vi "Tester.vi"() -> ()   [LabVIEW 2018, in "AE75TX Actor.lvlib" / "AE75TX.lvclass"]
uses:
  AE75TX.lvclass
  <vilib>/ORNL/CSEISMIC DDS/CSEISMIC DDS Base/Data Types/IED_Status.ctl
  <vilib>/ORNL/CSEISMIC DDS/CSEISMIC DDS Base/Data Types/Controls/DeviceID.ctl
  <vilib>/ORNL/CSEISMIC DDS/CSEISMIC DDS Base/Data Types/Controls/Timestamp.ctl
  <vilib>/ORNL/CSEISMIC DDS/CSEISMIC DDS Base/Data Types/DER_Measurement.ctl
  <vilib>/ORNL/CSEISMIC DDS/CSEISMIC DDS Base/Data Types/DER_Status.ctl
  <vilib>/ORNL/CSEISMIC DDS/CSEISMIC DDS Base/Data Types/Controls/DroopCurve.ctl
  Controls/PV State Selector.ctl
  Controls/Modbus Configuration Cluster.ctl
  Controls/Scaling Coefficients Measurements.ctl
  <vilib>/Modbus/master/Create Master Instance (TCP).vi
  <vilib>/Modbus/master/Modbus Master.lvclass
  <vilib>/ORNL/CSEISMIC DDS/CSEISMIC DDS Base/CSEISMIC DDS.lvclass
panel:
  in  "Ramp Rate (kVA/s)":u16
  in  "Curtailment (%)":u16
  in  "Write Curtailment":bool
  out "DER_Status":T1
  out "DER_Measurement":T4
  out "IED_Status":T5
  in  "stop":bool
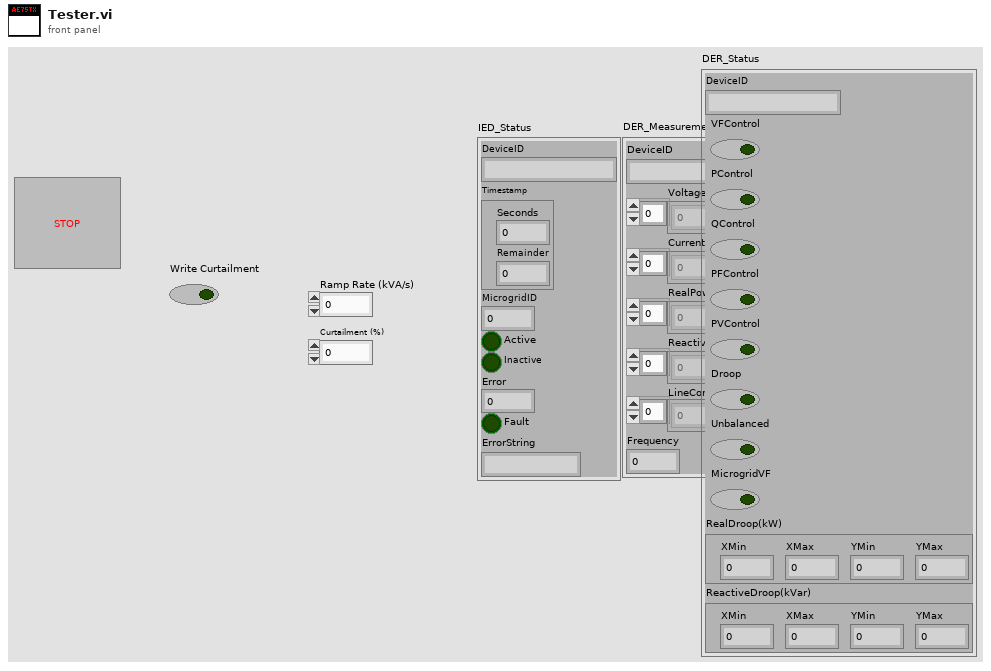
[diagram p1: front panel]
types:
  T1 = typedef "CSEISMIC DDS.lvlib/CSEISMIC DDS.lvclass/DER_Status.ctl" = cluster{"DeviceID":T2, "VFControl":bool, "PControl":bool, "QControl":bool, "PFControl":bool, "PVControl":bool, "Droop":bool, "Unbalanced":bool, "MicrogridVF":bool, "RealDroop(kW)":T3, "ReactiveDroop(kVar)":T3}
  T2 = typedef "CSEISMIC DDS.lvlib/CSEISMIC DDS.lvclass/DeviceID.ctl" = string
  T3 = typedef "CSEISMIC DDS.lvlib/CSEISMIC DDS.lvclass/DroopCurve.ctl" = cluster{"XMin":dbl, "XMax":dbl, "YMin":dbl, "YMax":dbl}
  T4 = typedef "CSEISMIC DDS.lvlib/CSEISMIC DDS.lvclass/DER_Measurement.ctl" = cluster{"DeviceID":T2, "Voltage":dbl[], "Current":dbl[], "RealPower":dbl[], "ReactivePower":dbl[], "LineConfig":u8[], "Frequency":dbl}
  T5 = typedef "CSEISMIC DDS.lvlib/CSEISMIC DDS.lvclass/IED_Status.ctl" = cluster{"DeviceID":T2, "Timestamp":T6, "MicrogridID":u8, "Active":bool, "Inactive":bool, "Error":i32, "Fault":bool, "ErrorString":string}
  T6 = typedef "CSEISMIC DDS.lvlib/CSEISMIC DDS.lvclass/Timestamp.ctl" = cluster{"Seconds":u64, "Remainder":u64}
  T7 = typedef "AE75TX Actor.lvlib/AE75TX.lvclass/Modbus Configuration Cluster.ctl" = cluster{"IP Address":string, "Port":u16, "DeviceID":T2}
  T8 = typedef "AE75TX Actor.lvlib/AE75TX.lvclass/PV State Selector.ctl" = enum16{"Init", "Read", "Error Check", "Close"}
  T9 = typedef "AE75TX Actor.lvlib/AE75TX.lvclass/Scaling Coefficients Measurements.ctl" = cluster{"Current":dbl, "Voltage":dbl, "Real Power":dbl, "Reactive Power":dbl, "Frequency":dbl}
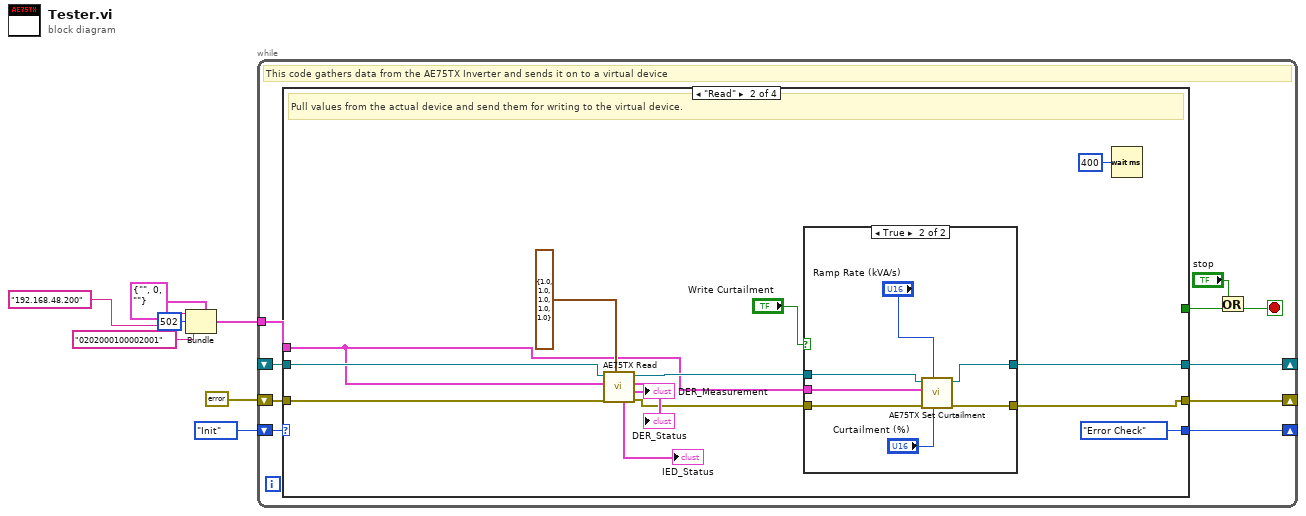
[diagram p0: block diagram]
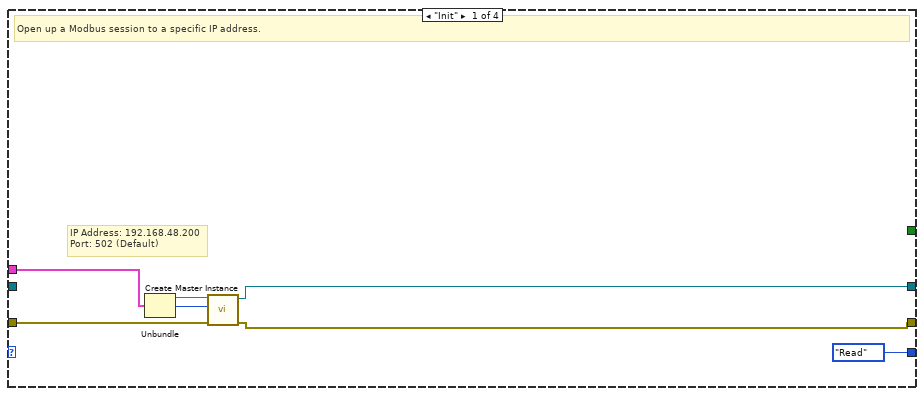
[diagram p2: hidden frame]
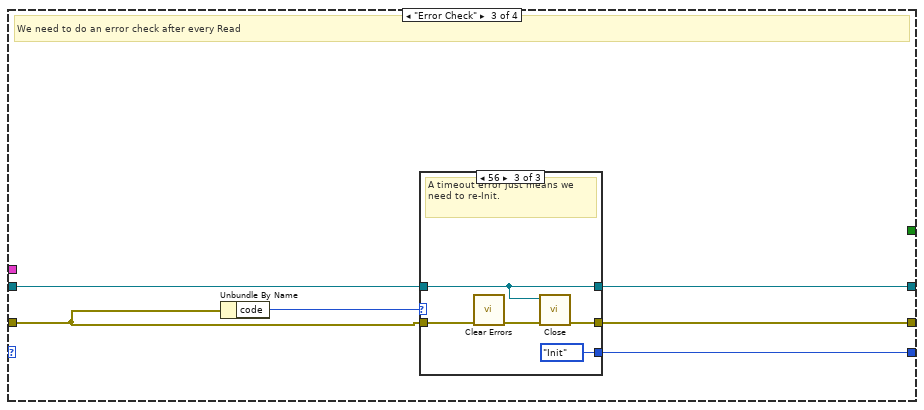
[diagram p4: hidden frame]
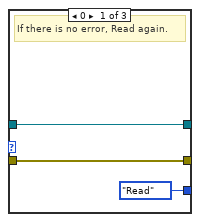
[diagram p5: hidden frame]
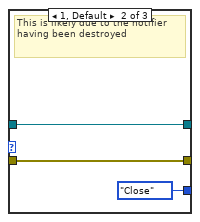
[diagram p6: hidden frame]
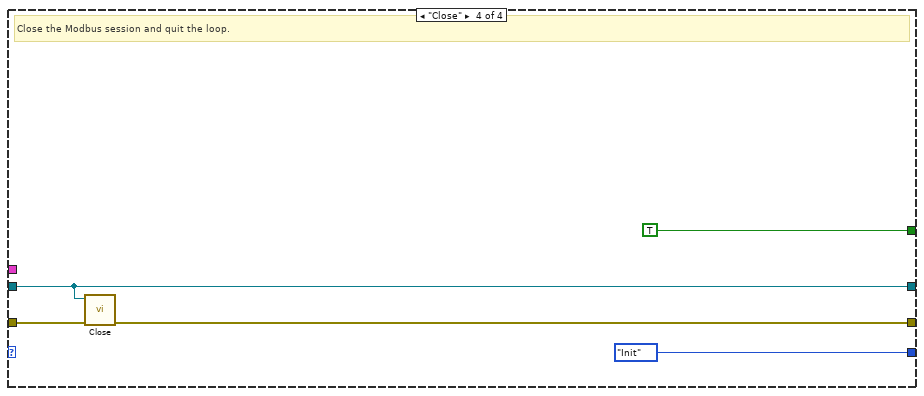
[diagram p7: hidden frame]
diagram:
  n1 = Bundle(cluster=T7 {"IP Address"="", "Port"=0, "DeviceID"=""} ("Modbus Configuration"), "IP Address"="192.168.48.200" ("address"), "Port"=u16 502, "DeviceID"=T2 "0202000100002001") -> (w1:T7)
  n2 = while {
    shift-right: [w15] -> _
    shift-left: PV_State_Selector."Init" -> [w17]
    shift-right: [w16] -> _
    shift-left: _ -> [w14]
    shift-right: [w12] -> _
    shift-left: errorcluster {"status"=FALSE, "code"=0, "source"=""} ("error out") -> [w13]
    tunnel: w1 -> [w8]
    stop <- w10 stop-if-true
    # "This code gathers data from the AE75TX Inverter and sends it on to a virtual device"
    n3 = case shown="\"Read\"" w17 {
      tunnel: [w19 w29 w49 w66] -> w16
      tunnel: [w18 w28 w52 w68] -> w12
      tunnel: [PV_State_Selector."Read" PV_State_Selector."Error Check" w50 PV_State_Selector."Init"] -> w15
      tunnel: w14 -> [_ w37 w51 w66]
      tunnel: w13 -> [w23 w36 w48 w69]
      tunnel: [_ _ _ TRUE ("stop")] -> w11
      tunnel: w8 -> [w22 w30 _ _]
      frame "Init" {
        # "IP Address: 192.168.48.200\nPort: 502 (Default)"
        # "Open up a Modbus session to a specific IP address."
        n4 = Unbundle(w22) -> ("IP Address"=w21:string, "Port"=w20:u16)  [unwired: 1 out]
        n5 = call-poly <vilib>:"Create Master Instance.vi"("error in (no error)"=w23, "port (502)"=w20, "address"=w21) -> ("error out"=w18:errorcluster, "TCP master instance"=w19:refnum<class "Modbus Master.lvclass">)  [unwired: 7 in]
      }
      frame "Read" {
        # "Pull values from the actual device and send them for writing to the virtual device."
        n6 = call "AE75TX Read.vi"("Scaling Coefficients"=T9 {"Current"=1.0, "Voltage"=1.0, "Real Power"=1.0, "Reactive Power"=1.0, "Frequency"=1.0}, "error in"=w36, "Modbus Configuration"=w30, "Modbus Master in"=w37) -> ("error out"=w31:errorcluster, "DER_Measurement"=→"DER_Measurement":T4, "DER_Status"=→"DER_Status":T1, "Modbus Master out"=w32:refnum<class "Modbus Master.lvclass">, "IED_Status"=→"IED_Status":T5)  [unwired: 3 in]
        n7 = case shown="True" "Write Curtailment" {
          tunnel: w32 -> [w40 w47]
          tunnel: w31 -> [w39 w46]
          tunnel: w30 -> [_ w45]
          tunnel: [w40 w44] -> w29
          tunnel: [w39 w43] -> w28
          frame False {
          }
          frame True {
            n8 = call "AE75TX Set Curtailment.vi"("Curtailment (%)"="Curtailment (%)", "Ramp Rate (kVA/s)"="Ramp Rate (kVA/s)", "error in"=w46, "Modbus Configuration"=w45, "Modbus Master in"=w47) -> ("error out"=w43:errorcluster, "Modbus Master out"=w44:refnum<class "Modbus Master.lvclass">)  [unwired: 5 in]
          }
        }
        n9 = Wait (ms)(milliseconds to wait=u32 400) -> ()  [unwired: 1 out]
      }
      frame "Error Check" {
        # "We need to do an error check after every Read"
        n10 = Unbundle By Name(w48) -> ("code"=w53:i32)
        n11 = case shown="56" w53 {
          tunnel: w48 -> [w56 w57 w64]
          tunnel: [w56 w57 w62] -> w52
          tunnel: w51 -> [w55 w58 w60]
          tunnel: [PV_State_Selector."Read" PV_State_Selector."Close" PV_State_Selector."Init"] -> w50
          tunnel: [w55 w58 w60] -> w49
          frame 0 {
            # "If there is no error, Read again."
          }
          frame 1, Default {
            # "This is likely due to the notifier having been destroyed"
          }
          frame 56 {
            # "A timeout error just means we need to re-Init."
            n12 = call <vilib>:"Clear Errors.vi"("error in (no error)"=w64) -> ("error out"=w63:errorcluster)  [unwired: 5 in, 1 out]
            n13 = call-dynamic "Close.vi"("error in (no error)"=w63, "Modbus master in"=w60) -> ("error out"=w62:errorcluster)  [unwired: 9 in]
          }
        }
      }
      frame "Close" {
        # "Close the Modbus session and quit the loop."
        n14 = call-dynamic "Close.vi"("error in (no error)"=w69, "Modbus master in"=w66) -> ("error out"=w68:errorcluster)  [unwired: 9 in]
      }
    }
    n15 = Or(x="stop", y=w11) -> (x .or. y?=w10:bool)
  }
